vi "PerformanceAnalizer.vi"() -> ()   [LabVIEW 2010]
uses:
  <vilib>/picture/picture.llb/Draw True-Color Pixmap.vi
  <vilib>/Utility/file.llb/Write To Spreadsheet File (DBL).vi
  <vilib>/Utility/file.llb/Write To Spreadsheet File (string).vi
panel:
  out "KTH  Automatic Control \nWireless Process Control over IEEE 802.15.4":picture
  in  "Tab Control":enum32{"Communication", "Configuration"}(tab)
  out "reliability =pckSuccess/pckTotal":dynamicdata(graph)
  out "errors":dynamicdata(graph)
  out "Inter sampling time = t_k - t_k-1":dynamicdata(graph)
  out "delay = t_send - t_ack":dynamicdata(graph)
  in  "StartSaving":bool
  in  "Saving":bool
  in  "StopSaving":bool
  out "Path":path
  out "errors_u":dbl
  out "errors_theta":dbl
  out "delay_xc":dbl
  out "delay_u":dbl
  out "delay_theta":dbl
  out "interSampling_xc":dbl
  out "interSampling_theta":dbl
  out "interSampling_u":dbl
  out "errors_xc":dbl
  out "reliability_u":dbl
  out "reliability_xc":dbl
  out "reliability_theta":dbl
  out "current time":timestamp
  out "Packet Window":i32=200
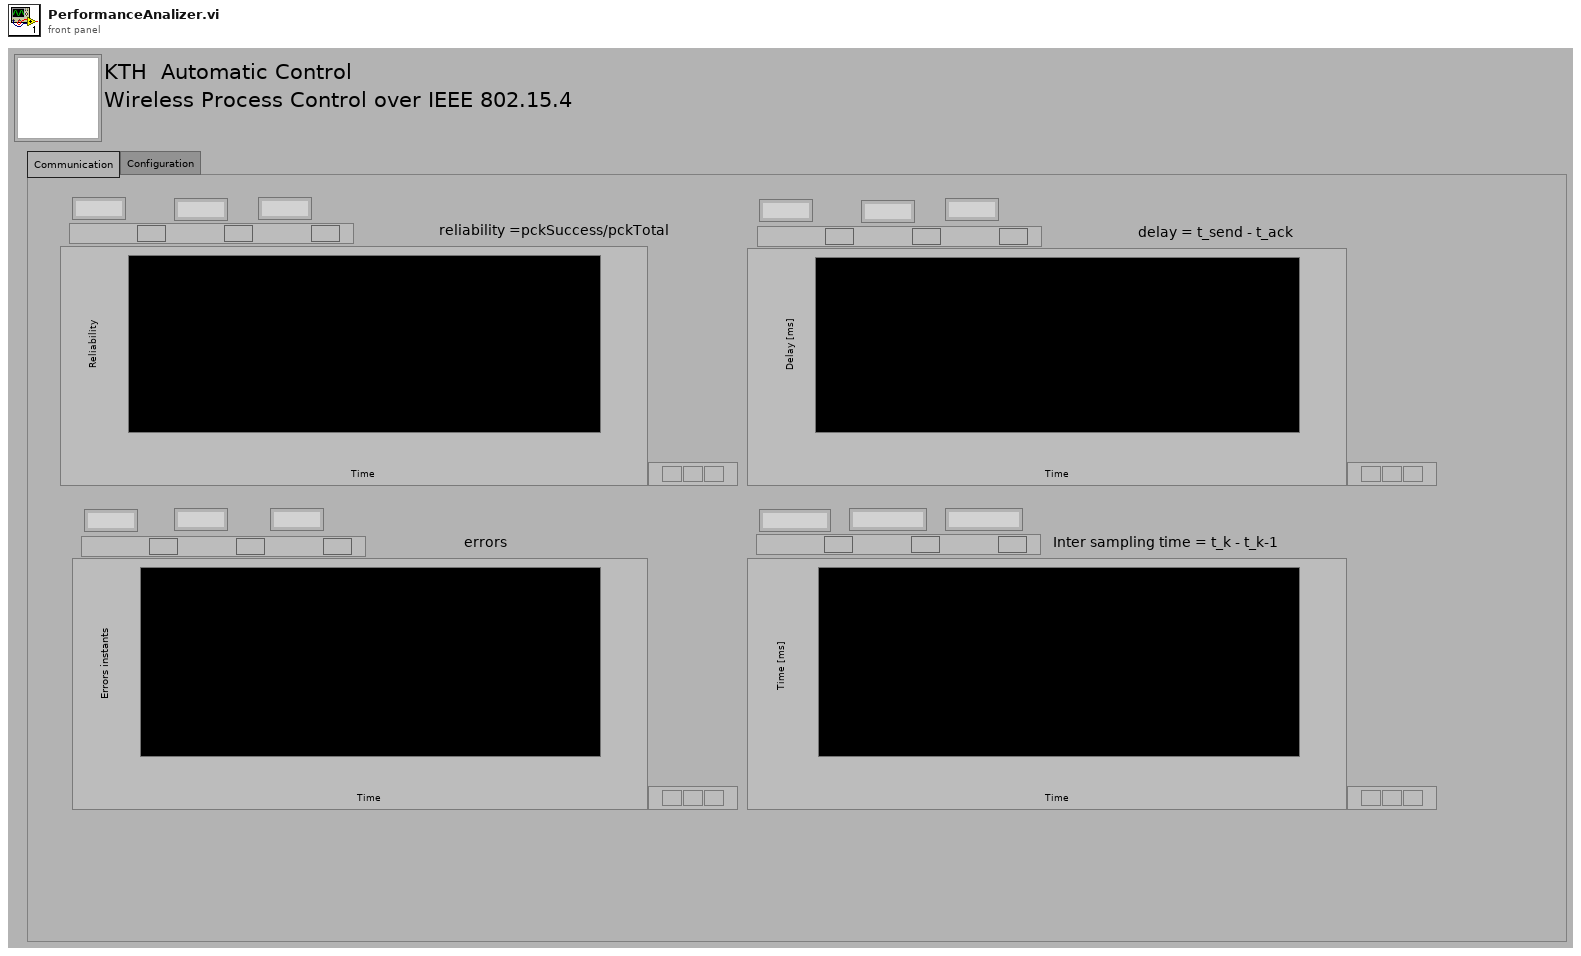
[diagram p1: front panel]
types:
  T1 = enum8{"Enabled", "Disabled", "Disabled and Grayed Out"}
  T2 = typedef "imagedata.ctl" = cluster{"image type":i32, "image depth":i32, "image":u8[], "mask":u8[], "colors":u32[], "Rectangle":cluster{"left":i16, "top":i16, "right":i16, "bottom":i16}}
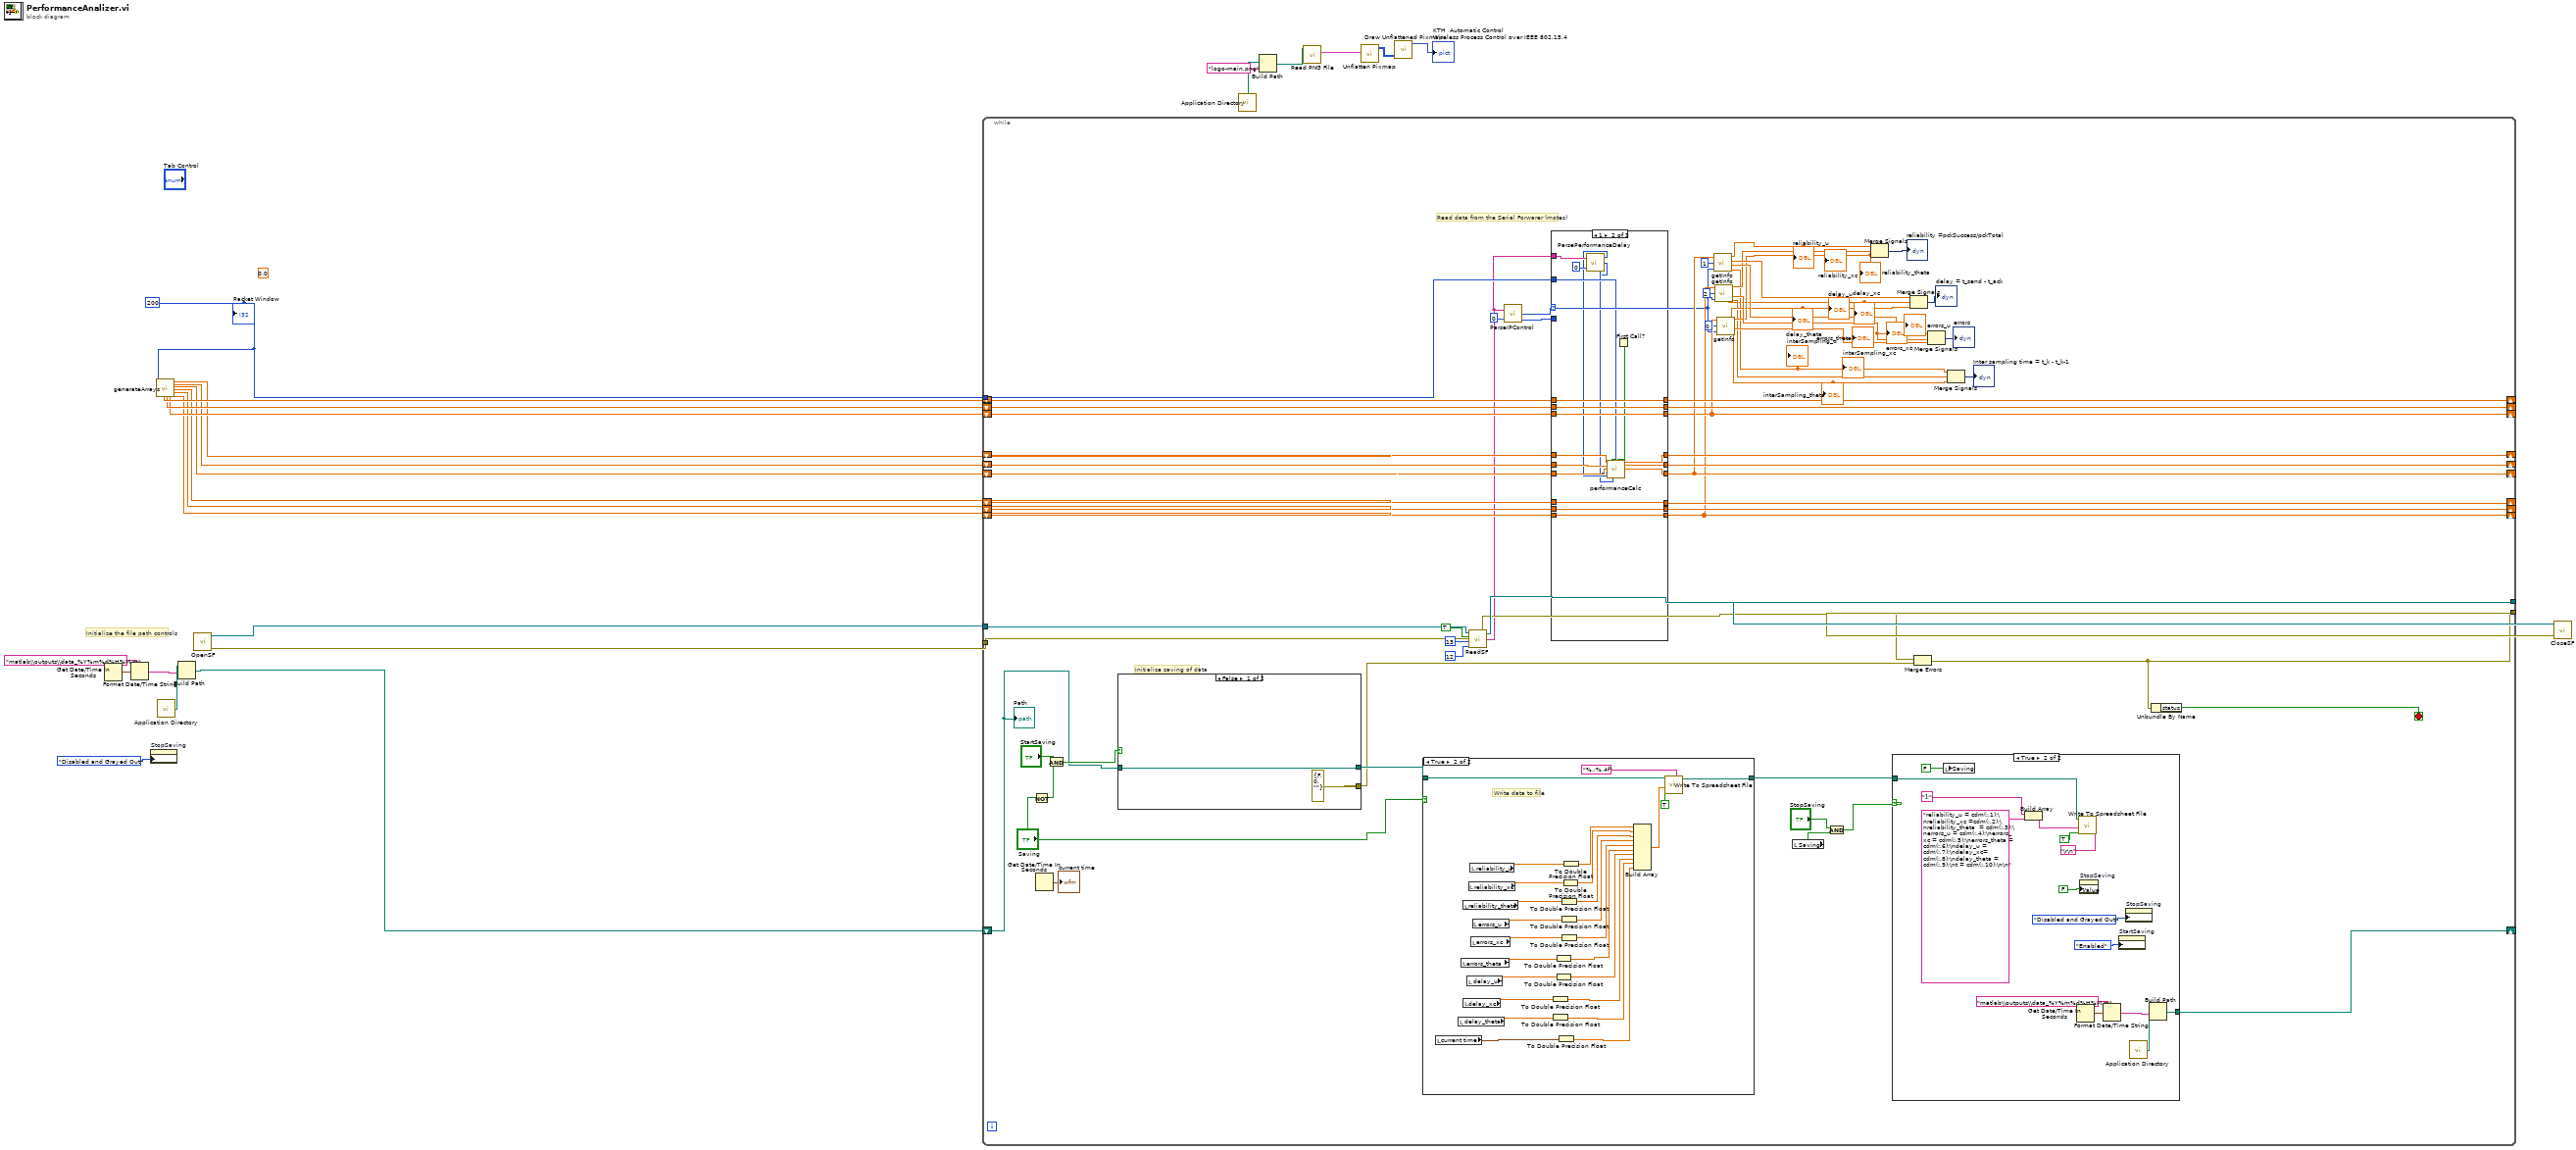
[diagram p0: block diagram]
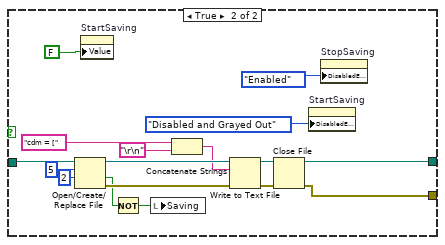
[diagram p4: hidden frame]
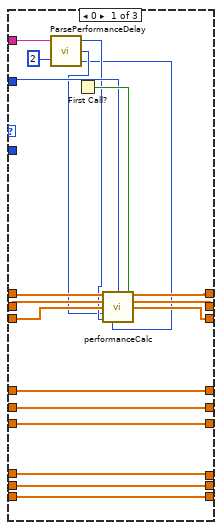
[diagram p5: hidden frame]
diagram:
  w23 = 200 ("Packet Window")
  (unwired) 0.0 ("prevPckTotalOut")
  # "Initialize the file path controls"
  n1 = Get Date/Time In Seconds() -> (seconds since 1Jan1904=w12:timestamp)
  n2 = Format Date/Time String(time format string (%c)="matlab\\outputs\\data_%Y%m%d%H%M.m", seconds (now)=w12) -> (date/time string=w10:string)  [unwired: 1 in]
  n3 = property on="StopSaving" class="Bool (strict)"("DisabledEnum"=T1."Disabled and Grayed Out" ("Disabled")) -> ()  [unwired: 2 in, 2 out]
  n4 = call "generateArrays.vi"("dimension size"=w23) -> ("errorsWindow1"=w22:dbl[], "pckTotalTrack1"=w21:dbl[], "state1"=w20:dbl[], "errorsWindow2"=w19:dbl[], "pckTotalTrack2"=w18:dbl[], "state2"=w17:dbl[], "errorsWindow3"=w16:dbl[], "pckTotalTrack3"=w15:dbl[], "state3"=w14:dbl[])  [unwired: 10 in]
  n5 = call <vilib>:"Application Directory.vi"() -> ("Application Directory"=w13:path)
  n6 = Build Path(base path=w13, name or relative path=w10) -> (appended path=w7:path)
  n7 = call "OpenSF.vi"() -> ("error out"=w25:errorcluster, "connection ID"=w26:refnum<k5>)  [unwired: 1 out]
  n8 = while {
    tunnel: w26 -> [w81]
    tunnel: w25 -> [w90]
    tunnel: [w80] -> w24
    tunnel: [w39] -> w9
    tunnel: w23 -> [w85]
    shift-right: [w78] -> _
    shift-left: w22 -> [w76]
    shift-right: [w77] -> _
    shift-left: w21 -> [w75]
    shift-right: [w54] -> _
    shift-left: w20 -> [w74]
    shift-right: [w70] -> _
    shift-left: w19 -> [w73]
    shift-right: [w69] -> _
    shift-left: w18 -> [w72]
    shift-right: [w56] -> _
    shift-left: w17 -> [w71]
    shift-right: [w65] -> _
    shift-left: w16 -> [w68]
    shift-right: [w55] -> _
    shift-left: w15 -> [w67]
    shift-right: [w53] -> _
    shift-left: w14 -> [w66]
    shift-right: [w30] -> _
    shift-left: w7 -> [w29]
    stop <- w38 stop-if-true
    # "Initialize saving of data"
    # "Read data from the Serial Forwarer (motes)"
    n9 = Not(x="Saving") -> (.not. x?=w35:bool)
    n10 = Get Date/Time In Seconds() -> (seconds since 1Jan1904=→"current time":timestamp)
    n11 = And(x="StartSaving", y=w35) -> (x .and. y?=w36:bool)
    n12 = case shown="False" w36 {
      tunnel: w29 -> [w134 w143]
      tunnel: [w134 w140] -> w45
      tunnel: [errorcluster {"status"=FALSE, "code"=0, "source"=""} ("error out") w137] -> w40
      frame False {
      }
      frame True {
        n13 = Open/Create/Replace File(file path (use dialog)=w143, operation (0:open)=5, access (0:read/write)=2) -> (refnum out=w149:refnum<file>, cancelled=w142:bool, error out=w146:errorcluster)  [unwired: 3 in]
        n14 = property on="StartSaving" class="Bool (strict)"("Value"=FALSE ("StartSaving")) -> ()  [unwired: 2 in, 2 out]
        n15 = Not(x=w142) -> (.not. x?=w139:bool)
        n16 = local write "Saving"(w139) -> ()
        n17 = Concatenate Strings("cdm = [", "\r\n") -> (w145:string)
        n18 = Write to Text File(file (use dialog)=w149, text=w145, error in=w146) -> (refnum out=w148:refnum<file>, error out=w147:errorcluster)  [unwired: 1 in, 1 out]
        n19 = Close File(refnum=w148, error in=w147) -> (path=w140:path, error out=w137:errorcluster)
        n20 = property on="StartSaving" class="Bool (strict)"("DisabledEnum"=T1."Disabled and Grayed Out" ("Disabled")) -> ()  [unwired: 2 in, 2 out]
        n21 = property on="StopSaving" class="Bool (strict)"("DisabledEnum"=T1."Enabled" ("Disabled")) -> ()  [unwired: 2 in, 2 out]
      }
    }
    n22 = case shown="True" "Saving" {
      tunnel: w45 -> [w107 w131]
      tunnel: [w107 w108] -> w42
      frame False {
      }
      frame True {
        # "Write data to file"
        n23 = local read "current time"() -> (w109:timestamp)
        n24 = local read "delay_theta"() -> (w117:dbl)
        n25 = local read "errors_theta"() -> (w118:dbl)
        n26 = local read "reliability_theta"() -> (w126:dbl)
        n27 = local read "delay_xc"() -> (w116:dbl)
        n28 = local read "delay_u"() -> (w119:dbl)
        n29 = local read "reliability_xc"() -> (w127:dbl)
        n30 = local read "reliability_u"() -> (w129:dbl)
        n31 = local read "errors_xc"() -> (w122:dbl)
        n32 = local read "errors_u"() -> (w125:dbl)
        n33 = To Double Precision Float(number=w116) -> (double precision float=w113:dbl)
        n34 = To Double Precision Float(number=w117) -> (double precision float=w112:dbl)
        n35 = To Double Precision Float(number=w118) -> (double precision float=w115:dbl)
        n36 = To Double Precision Float(number=w119) -> (double precision float=w114:dbl)
        n37 = To Double Precision Float(number=w109) -> (double precision float=w110:dbl)
        n38 = To Double Precision Float(number=w126) -> (double precision float=w123:dbl)
        n39 = To Double Precision Float(number=w125) -> (double precision float=w121:dbl)
        n40 = To Double Precision Float(number=w122) -> (double precision float=w120:dbl)
        n41 = To Double Precision Float(number=w127) -> (double precision float=w124:dbl)
        n42 = To Double Precision Float(number=w129) -> (double precision float=w128:dbl)
        n43 = Build Array(w128, w124, w123, w121, w120, w115, w114, w113, w112, w110) -> (w111:dbl[])
        n44 = call-poly <vilib>:"Write To Spreadsheet File.vi"("format (%.3f)"="%.;%.4f", "append to file? (new file:F)"=TRUE, "1D data"=w111, "file path (dialog if empty)"=w131) -> ("new file path (Not A Path if cancelled)"=w108:path)  [unwired: 4 in]
      }
    }
    n45 = call "ReadSF.vi"("connection ID in"=w81, "enabled"=TRUE, "bytes to read"=13 ("f"), "header size"=12 ("bytes to read"), "error in"=w90) -> ("connection ID out"=w80:refnum<k5>, "string"=w28:string, "error out"=w41:errorcluster)
    n46 = call "ParseIPControl.vi"("data out"=w28, "offset"=u8 0) -> ("srcId"=w27:u8, "data"=w82:i16)  [unwired: 1 in]
    n47 = case shown="1" w27 {
      tunnel: w82 -> [_ _ _]
      tunnel: w85 -> [w169 w180 _]
      tunnel: [w165 w189 w198] -> w78
      tunnel: [w164 w188 w197] -> w77
      tunnel: [w163 w187 w196] -> w54
      tunnel: w76 -> [w168 w189 w198]
      tunnel: w75 -> [w167 w188 w197]
      tunnel: w74 -> [w166 w187 w196]
      tunnel: w73 -> [w162 w183 w195]
      tunnel: w72 -> [w161 w182 w194]
      tunnel: w71 -> [w160 w181 w193]
      tunnel: [w162 w179 w195] -> w70
      tunnel: [w161 w178 w194] -> w69
      tunnel: [w160 w177 w193] -> w56
      tunnel: w68 -> [w159 w186 w192]
      tunnel: w67 -> [w158 w185 w191]
      tunnel: w66 -> [w157 w184 w190]
      tunnel: [w159 w186 w192] -> w65
      tunnel: [w158 w185 w191] -> w55
      tunnel: [w157 w184 w190] -> w53
      tunnel: w28 -> [w155 w175 _]
      frame 0 {
        n48 = call "ParsePerformanceDelay.vi"("data out"=w155, "offset"=2) -> ("pckTotal"=w154:u16, "pckSuccess"=w153:u16, "delay"=w152:u16)
        n49 = First Call?() -> (First Call?: T/F=w170:bool)
        n50 = call "performanceCalc.vi"("errors"=w168, "init"=w170, "windowLength"=w169, "pckTotalTrack"=w167, "state"=w166, "pckSuccess"=w153, "pckTotal"=w154, "delay"=w152) -> ("errorsOut"=w165:dbl[], "pckTotalTrackOut"=w164:dbl[], "prevState"=w163:dbl[])  [unwired: 5 in]
      }
      frame 1 {
        n51 = call "ParsePerformanceDelay.vi"("data out"=w175, "offset"=0) -> ("pckTotal"=w173:u16, "pckSuccess"=w171:u16, "delay"=w172:u16)
        n52 = First Call?() -> (First Call?: T/F=w176:bool)
        n53 = call "performanceCalc.vi"("errors"=w183, "init"=w176, "windowLength"=w180, "pckTotalTrack"=w182, "state"=w181, "pckSuccess"=w171, "pckTotal"=w173, "delay"=w172) -> ("errorsOut"=w179:dbl[], "pckTotalTrackOut"=w178:dbl[], "prevState"=w177:dbl[])  [unwired: 5 in]
      }
      frame 3, Default {
      }
    }
    n54 = call "getInfo.vi"("array"=w56, "srcID"=u16 1, "srcIDPck"=w27) -> ("reliability"=w64:dbl, "delay"=w63:dbl, "errors"=w62:dbl, "interSampling"=w48:dbl)
    "reliability_u" <- w64
    "errors_u" <- w62
    "interSampling_u" <- w48
    "delay_u" <- w63
    n55 = call "getInfo.vi"("array"=w53, "srcID"=u16 2, "srcIDPck"=w27) -> ("reliability"=w61:dbl, "delay"=w44:dbl, "errors"=w60:dbl, "interSampling"=w47:dbl)
    "reliability_xc" <- w61
    "errors_xc" <- w60
    "interSampling_xc" <- w47
    "delay_xc" <- w44
    n56 = call "getInfo.vi"("array"=w54, "srcID"=u16 0, "srcIDPck"=w27) -> ("reliability"=w59:dbl, "delay"=w58:dbl, "errors"=w57:dbl, "interSampling"=w46:dbl)
    "reliability_theta" <- w59
    "errors_theta" <- w57
    "interSampling_theta" <- w46
    "delay_theta" <- w58
    n57 = local read "Saving"() -> (w31:bool)
    n58 = And(x="StopSaving", y=w31) -> (x .and. y?=w32:bool)
    n59 = Merge Signals(w64, w61, w59) -> (→"reliability =pckSuccess/pckTotal":dynamicdata)
    n60 = case shown="True" w32 {
      tunnel: w42 -> [w91 w99]
      tunnel: [w91 w92] -> w30
      frame False {
      }
      frame True {
        n61 = local write "Saving"(FALSE) -> ()
        n62 = Build Array("];", "reliability_u = cdm(:,1);\nreliability_xc =cdm(:,2);\nreliability_theta  = cdm(:,3);\nerrors_u = cdm(:,4);\nerrors_xc = cdm(:,5);\nerrors_theta = cdm(:,6);\ndelay_u = cdm(:,7);\ndelay_xc= cdm(:,8);\ndelay_theta = cdm(:,9);\nt = cdm(:,10);\n\n") -> (w104:string[])
        n63 = Get Date/Time In Seconds() -> (seconds since 1Jan1904=w95:timestamp)
        n64 = call-poly <vilib>:"Write To Spreadsheet File.vi"("delimiter (\\t)"="\r\n", "append to file? (new file:F)"=TRUE, "1D data"=w104, "file path (dialog if empty)"=w99) -> ()  [unwired: 4 in, 1 out]
        n65 = property on="StopSaving" class="Bool (strict)"("Value"=FALSE ("StartSaving")) -> ()  [unwired: 2 in, 2 out]
        n66 = Format Date/Time String(time format string (%c)="matlab\\outputs\\data_%Y%m%d%H%M.m", seconds (now)=w95) -> (date/time string=w93:string)  [unwired: 1 in]
        n67 = property on="StartSaving" class="Bool (strict)"("DisabledEnum"=T1."Enabled" ("Disabled")) -> ()  [unwired: 2 in, 2 out]
        n68 = property on="StopSaving" class="Bool (strict)"("DisabledEnum"=T1."Disabled and Grayed Out" ("Disabled")) -> ()  [unwired: 2 in, 2 out]
        n69 = call <vilib>:"Application Directory.vi"() -> ("Application Directory"=w96:path)
        n70 = Build Path(base path=w96, name or relative path=w93) -> (appended path=w92:path)
      }
    }
    n71 = Merge Signals(w63, w44, w58) -> (→"delay = t_send - t_ack":dynamicdata)
    n72 = Merge Errors(w41, w40) -> (w39:errorcluster)
    n73 = Merge Signals(w62, w60, w57) -> (→"errors":dynamicdata)
    n74 = Merge Signals(w48, w47, w46) -> (→"Inter sampling time = t_k - t_k-1":dynamicdata)
    n75 = Unbundle By Name(w39) -> ("status"=w38:bool)
    "Path" <- w29
  }
  n76 = call <vilib>:"Application Directory.vi"() -> ("Application Directory"=w2:path)
  n77 = Build Path(base path=w2, name or relative path="logo-main.png") -> (appended path=w3:path)
  n78 = call <vilib>:"Read PNG File.vi"("path to PNG file"=w3) -> ("image data"=w6:T2)  [unwired: 8 in, 2 out]
  n79 = call <vilib>:"Unflatten Pixmap.vi"("image data"=w6) -> ("24-bit pixmap"=w5:u32[][])  [unwired: 4 in, 6 out]
  n80 = call-poly <vilib>:"Draw Unflattened Pixmap.vi"("data (RGB format)"=w5) -> ("new picture"=→"KTH  Automatic Control \nWireless Process Control over IEEE 802.15.4":picture)  [unwired: 8 in]
  n81 = call "CloseSF.vi"("error out"=w9, "connection ID"=w24) -> ()  [unwired: 1 in]
  "Packet Window" <- w23
